vi "Read Accelerometer Values And Write to Serial.vi"() -> ()   [LabVIEW 2014]
doc: "Tested on:\n - Arduino Nano\n - WemosD1 with ESP8266\n\nSending raw accelerometer data through UART to computer."
uses:
  <vilib>/LabVIEW Universal Transcriptor/LabVIEW to Arduino Transcriptor/Transcriptors/System API/Serial println string.vi
  <vilib>/LabVIEW Universal Transcriptor/Arduino MPU6050 Library/Arduino MPU6050.lvlib
panel:
  in  "serial speed (Bd)":i32=115200
  in  "address":u16(ring)=104 items=["AD0 pin NOT CONNECTED"=104, "AD0 connect to Vcc"=105]
  in  "range":T1(ring)
  in  "scale":T2(ring)
  in  "Error In":errorcluster
  out "error out":errorcluster
  # "Wiring:\nMPU6050 | WemosD1 | Arduino\n        |         | Nano\n--------+---------+----------\nVcc     | +5V     | +5V\nGND     | GND     | GND\nSCL     | D15/SCL | A5\nSDA     | D14/SCA | A4\nSCA     | D14/SDA"
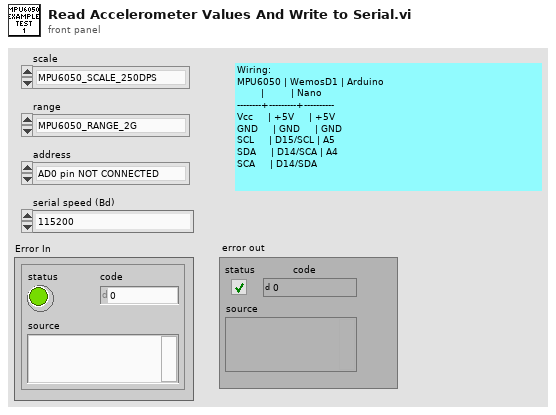
[diagram p1: front panel]
types:
  T1 = enum16{"MPU6050_RANGE_2G", "MPU6050_RANGE_4G", "MPU6050_RANGE_8G", "MPU6050_RANGE_16G"}
  T2 = enum16{"MPU6050_SCALE_250DPS", "MPU6050_SCALE_500DPS", "MPU6050_SCALE_1000DPS", "MPU6050_SCALE_2000DPS"}
  T3 = typedef "Arduino MPU6050.lvlib/MPU6050LibVector.ctl" = cluster{"XAxis":sgl, "YAxis":sgl, "ZAxis":sgl}
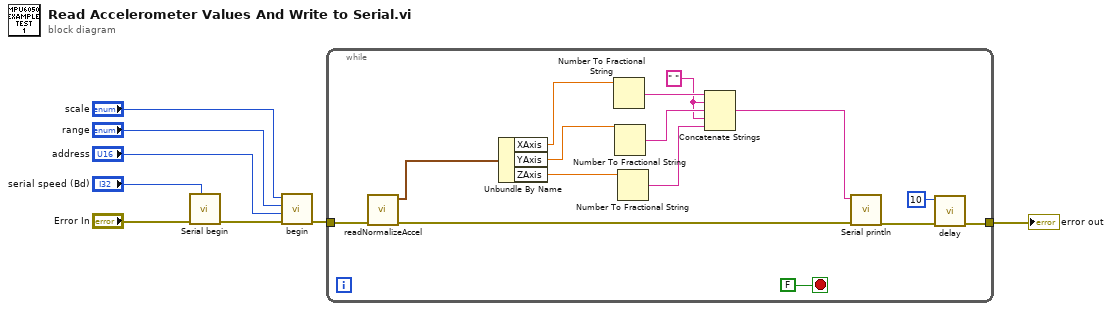
[diagram p0: block diagram]
diagram:
  n1 = call <vilib>:"Serial begin.vi"("Error In"="Error In", "speed (Bd)"="serial speed (Bd)") -> ("Error Out"=w7:errorcluster)  [unwired: 9 in]
  n2 = call <vilib>:"begin.vi"("Error In"=w7, "address"="address", "range"="range", "scale"="scale") -> ("Error Out"=w1:errorcluster)  [unwired: 7 in]
  n3 = while {
    tunnel: w1 -> [w11]
    tunnel: [w19] -> w8
    stop <- FALSE stop-if-true
    w12 = " " ("F-format string")
    n4 = call <vilib>:"readNormalizeAccel.vi"("error in (no error)"=w11) -> ("error out"=w10:errorcluster, "Vector"=w9:T3)  [unwired: 9 in]
    n5 = Unbundle By Name(w9) -> ("XAxis"=w22:sgl, "YAxis"=w21:sgl, "ZAxis"=w20:sgl)
    n6 = Number To Fractional String(number=w22) -> (F-format string=w16:string)  [unwired: 3 in]
    n7 = Number To Fractional String(number=w21) -> (F-format string=w15:string)  [unwired: 3 in]
    n8 = Number To Fractional String(number=w20) -> (F-format string=w14:string)  [unwired: 3 in]
    n9 = Concatenate Strings(w16, w12, w15, w12, w14) -> (w13:string)
    n10 = call-poly <vilib>:"Serial println.vi"("Error In"=w10, "string in"=w13) -> ("Error Out"=w18:errorcluster)  [unwired: 9 in]
    n11 = call <vilib>:"delay.vi"("Error In"=w18, "time (ms)"=10) -> ("Error Out"=w19:errorcluster)  [unwired: 9 in]
  }
  "error out" <- w8
